vi "Close.vi"(8 "Error In":errorcluster, 11 "ChipKit Configuration":T1={"COM Port"="", "Board Type"=enum."ChipKit Uno32", "Connection Type"=enum."USB / Serial", "Baud Rate (115200)"=15, "Bytes Per Packet (15)"=15}) -> (0 "Error Out":errorcluster)   [LabVIEW 2011, in "LabVIEW Interface for ChipKit.lvlib"]
doc: "Closes the connection to the ChipKit."
uses:
  LabVIEW Interface for ChipKit.lvlib
  Private/Type Defs/Chipkit Resource.ctl
  Private/Type Defs/Board Type.ctl
  Private/Type Defs/Connection Type.ctl
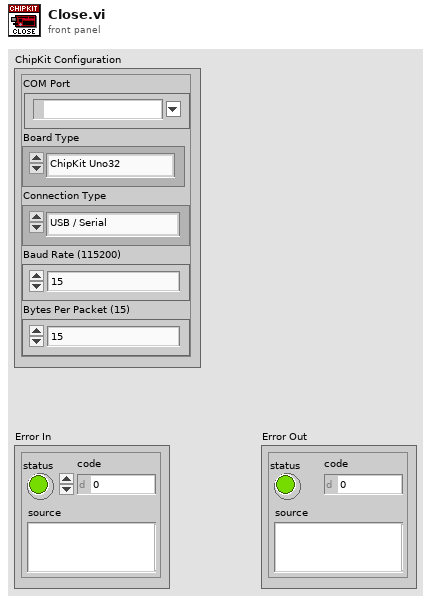
[diagram p1: front panel]
types:
  T1 = typedef "LabVIEW Interface for ChipKit.lvlib/Chipkit Resource.ctl" = cluster{"COM Port":refnum<visa-resource-name>, "Board Type":T2, "Connection Type":T3, "Baud Rate (115200)":u32, "Bytes Per Packet (15)":u32}
  T2 = typedef "LabVIEW Interface for ChipKit.lvlib/Board Type.ctl" = enum16{"ChipKit uC32", "ChipKit Uno32", "ChipKit Max32"}
  T3 = typedef "LabVIEW Interface for ChipKit.lvlib/Connection Type.ctl" = enum8{"USB / Serial", "XBEE", "BlueSmirf (Bluetooth)"}
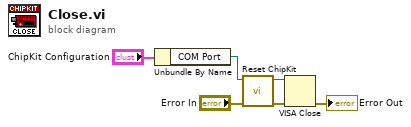
[diagram p0: block diagram]
diagram:
  n1 = Unbundle By Name("ChipKit Configuration") -> ("COM Port"=w5:refnum<visa-resource-name>)
  n2 = call "Reset ChipKit.vi"("Error In"="Error In", "VISA resource"=w5) -> ("Error Out"=w3:errorcluster, "VISA resource"=w1:refnum<visa-resource-name>)  [unwired: 8 in]
  n3 = VISA Close(VISA resource name=w1, error in (no error)=w3) -> (error out=→"Error Out":errorcluster)
